vi "8_1DArray(170382,170307).vi"() -> ()   [LabVIEW 2015]
panel:
  out "Max":dbl
  out "Min":dbl
  out "descending array":dbl[](array[numeric])
  out "Ascending array":dbl[](array[numeric])
  out "reversed array":dbl[](array[numeric])
  out "size(s)":i32
  in  "Array":dbl[](array[numeric])
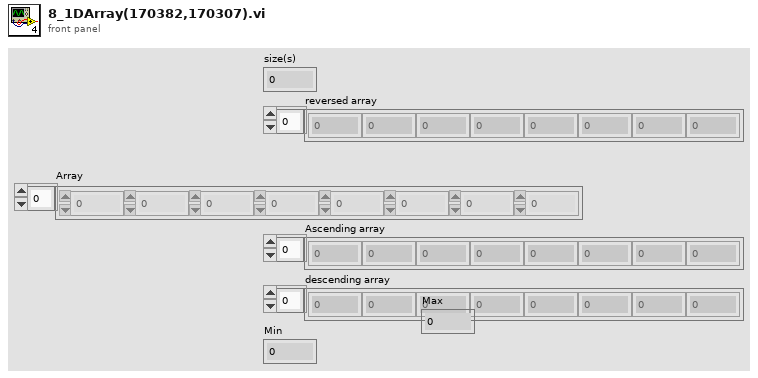
[diagram p1: front panel]
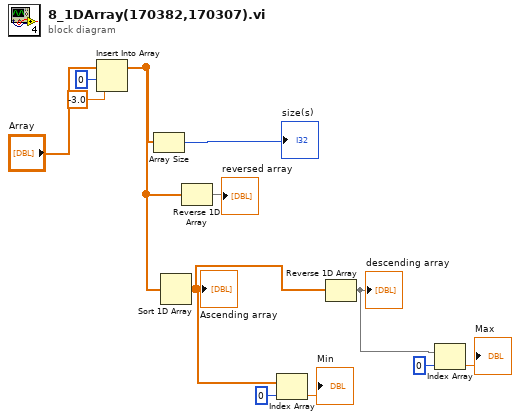
[diagram p0: block diagram]
diagram:
  n1 = Insert Into Array(array="Array", index=0, new element=-3.0 ("new element/subarray")) -> (w7:dbl[])
  n2 = Array Size(array=w7) -> (size(s)=→"size(s)":i32)
  n3 = Sort 1D Array(array=w7) -> (sorted array=w6:dbl[])
  "Ascending array" <- w6
  n4 = Reverse 1D Array(array=w7) -> (reversed array=→"reversed array":dbl[])
  n5 = Index Array(array=w6, index=0) -> (element=→"Min":dbl)
  n6 = Reverse 1D Array(array=w6) -> (reversed array=w1:dbl[])
  "descending array" <- w1
  n7 = Index Array(array=w1, index=0) -> (element=→"Max":dbl)
